vi "SortChannels.vi"(0 "DisplayTetrodes in":refnum<class "DisplayTetrodes.lvclass">, 11 "error in (no error)":errorcluster) -> (1 "sortedTetChanNum":i32[](array[numeric]), 3 "sortedTetNum":i32[](array[numeric]), 4 "DisplayTetrodes out":refnum<class "DisplayTetrodes.lvclass">, 6 "reorderedChanNums":i32[](array[numeric]), 10 "sortedChanIdx":i32[](array[numeric]), 12 "unsortedTetNums":i32[](array[numeric]), 13 "reorderedDiodeChan":i32, 15 "error out":errorcluster)   [LabVIEW 2010, in "DisplayTetrodes.lvclass"]
uses:
  DisplayTetrodes.lvclass
  <vilib>/regexp/Match Regular Expression.xnode
  <vilib>/imath/engines/lvmath2/RunTimeEngine/ErrorHandling/NIMS_Finalize Error.vi
  <vilib>/imath/engines/lvmath2/RunTimeEngine/NodeEndStatement/NIMS_NodeEndStatement_Output.vi
  <instcachedir>/0/NIMS_NodeEndStatement_Output_53EC0D466D134D7ABD903AC30B43404B.lvgen/NIMS_NodeEndStatement_Output_53EC0D466D134D7ABD903AC30B43404B_004.vi
  <instcachedir>/0/NIMS_NodeEndStatement_Output_53EC0D466D134D7ABD903AC30B43404B.lvgen/NIMS_NodeEndStatement_Output_53EC0D466D134D7ABD903AC30B43404B_005.vi
  <instcachedir>/0/NIMS_NodeEndStatement_Output_53EC0D466D134D7ABD903AC30B43404B.lvgen/NIMS_NodeEndStatement_Output_53EC0D466D134D7ABD903AC30B43404B_001.vi
  <vilib>/imath/engines/lvmath2/RunTimeEngine/VariableToken/Read/NIMS_Get Elements - RV(_) - Check(_).vi
  <instcachedir>/0/NIMS_Get Elements - RV(_) - Check(_)_260A45C9C4AF472A8F32F86A1BEF7DEE.lvgen/NIMS_Get Elements - RV(_) - Check(_)_260A45C9C4AF472A8F32F86A1BEF7DEE_001.vi
  <vilib>/imathl/engines/lvmath/Functions/Error Handling/Create Error.vi
  <vilib>/imath/engines/lvmath2/RunTimeEngine/BuiltInFunctions/sort/NIMS_[2o]_sort(RRowV,I32,Str).vi
  <instcachedir>/0/NIMS_[2o]_sort(RRowV,I32,Str)_1834406CABAC430BB40FEC772A4FC192.lvgen/NIMS_[2o]_sort(RRowV,I32,Str)_1834406CABAC430BB40FEC772A4FC192_001.vi
  <vilib>/imath/engines/lvmath2/RunTimeEngine/VariableToken/Read/NIMS_Get Elements - RV(_) - Check.vi
  <instcachedir>/0/NIMS_Get Elements - RV(_) - Check_1F6F8656162345078B1D4DC9877DFAE9.lvgen/NIMS_Get Elements - RV(_) - Check_1F6F8656162345078B1D4DC9877DFAE9_003.vi
  <vilib>/imath/engines/lvmath2/RunTimeEngine/BuiltInFunctions/length/NIMS_length(GV).vi
  <instcachedir>/0/NIMS_length(GV)_08A3D13377FD4E4B96F5795FBF3698FA.lvgen/NIMS_length(GV)_08A3D13377FD4E4B96F5795FBF3698FA_002.vi
  <vilib>/imath/engines/lvmath2/RunTimeEngine/ReplaceToken/NIMS_Replace - Check Linear.vi
  <instcachedir>/0/NIMS_Replace - Check Linear_662D5651E4E34E0584DA82A256193A4C.lvgen/NIMS_Replace - Check Linear_662D5651E4E34E0584DA82A256193A4C_007.vi
  <vilib>/imath/engines/lvmath2/RunTimeEngine/RangeToken/NIMS_Range.vi
  <instcachedir>/0/NIMS_Range_1C63927E4E474DADACDA97C3F2261A11.lvgen/NIMS_Range_1C63927E4E474DADACDA97C3F2261A11_000.vi
  <vilib>/imath/engines/lvmath2/RunTimeEngine/ReplaceToken/NIMS_Replace - Size Check _(_)=VorM.vi
  <instcachedir>/0/NIMS_Replace - Size Check _(_)=VorM_4228B35EE910471DB74F3866D9D09B95.lvgen/NIMS_Replace - Size Check _(_)=VorM_4228B35EE910471DB74F3866D9D09B95_007.vi
  <vilib>/imath/engines/lvmath2/RunTimeEngine/ReplaceToken/NIMS_Replace - Assignment Check _(_)=VorM.vi
  <instcachedir>/0/NIMS_Replace - Assignment Check _(_)=VorM_C130F3B8B64B4DD7B9359A2D3A035D18.lvgen/NIMS_Replace - Assignment Check _(_)=VorM_C130F3B8B64B4DD7B9359A2D3A035D18_007.vi
  <vilib>/imath/engines/lvmath2/RunTimeEngine/ErrorHandling/NIMS_Create Error From Enums.vi
  <vilib>/imath/engines/lvmath2/RunTimeEngine/BuiltInFunctions/findnz/NIMS_[1o]_findnz(GRowV).vi
  <instcachedir>/0/NIMS_[1o]_findnz(GRowV)_005A6E28988F485CA06F579662DA62C7.lvgen/NIMS_[1o]_findnz(GRowV)_005A6E28988F485CA06F579662DA62C7_002.vi
  <vilib>/imath/engines/lvmath2/RunTimeEngine/BuiltInFunctions/is_empty/NIMS_is_empty(GV).vi
  <instcachedir>/0/NIMS_is_empty(GV)_FC7E7C3D9544432CB6AA2416ADCF6D56.lvgen/NIMS_is_empty(GV)_FC7E7C3D9544432CB6AA2416ADCF6D56_000.vi
panel:
  out "size(s) 2":i32
  out "size(s)":i32
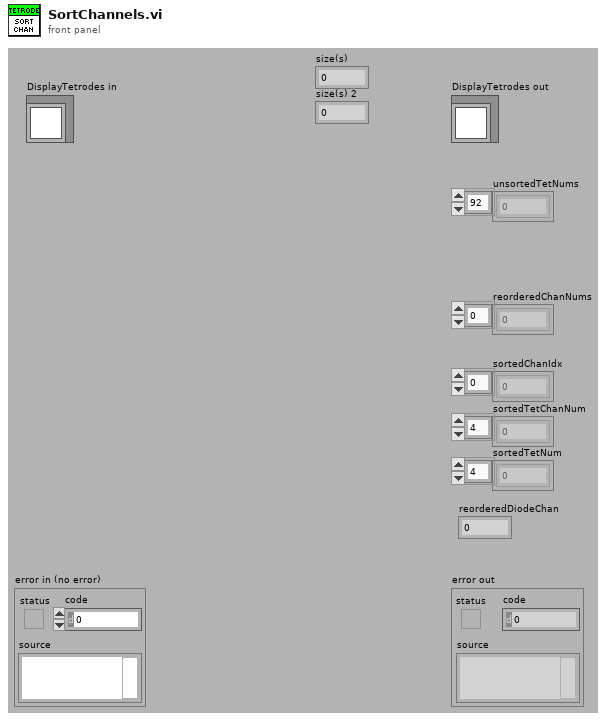
[diagram p1: front panel]
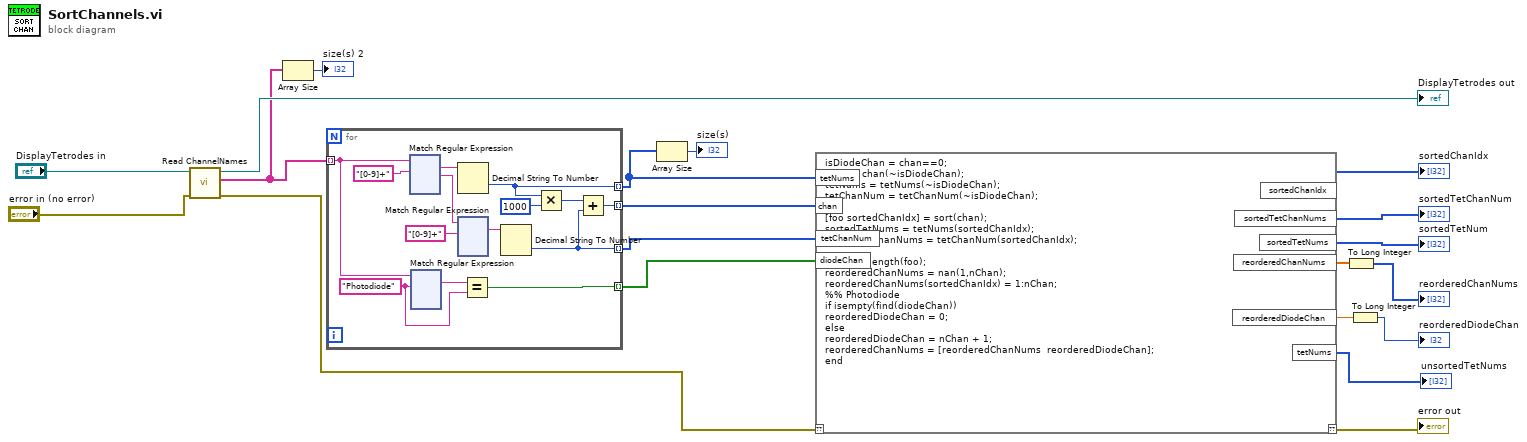
[diagram p0: block diagram]
diagram:
  n1 = call-dynamic "Read ChannelNames.vi"("error in (no error)"="error in (no error)", "DataReceiver in"="DisplayTetrodes in") -> ("error out"=w10:errorcluster, "ChannelNames"=w3:string[], "DataReceiver out"=→"DisplayTetrodes out":refnum<class "DisplayTetrodes.lvclass">)  [unwired: 7 in]
  n2 = Array Size(array=w3) -> (size(s)=→"size(s) 2":i32)
  n3 = for {
    tunnel: w3 -> [w25] mode=indexing
    tunnel: [w22] -> w19 mode=indexing
    tunnel: [w27] -> w5 mode=indexing
    tunnel: [w26] -> w20 mode=indexing
    tunnel: [w21] -> w8 mode=indexing
    w23 = "Photodiode" ("regular expression")
    n4 = xnode "Match Regular Expression"("input string"=w25, "regular expression"="[0-9]+") -> ("whole match"=w31:string, "after match"=w32:string)  [unwired: 4 in, 3 out]
    n5 = xnode "Match Regular Expression"("input string"=w25, "regular expression"=w23) -> ("whole match"=w24:string)  [unwired: 4 in, 4 out]
    n6 = Decimal String To Number(string=w31) -> (number=w27:i32)  [unwired: 2 in, 1 out]
    n7 = xnode "Match Regular Expression"("input string"=w32, "regular expression"="[0-9]+") -> ("whole match"=w30:string)  [unwired: 4 in, 4 out]
    n8 = Equal?(x=w24, y=w23) -> (x = y?=w21:bool)
    n9 = Decimal String To Number(string=w30) -> (number=w26:i32)  [unwired: 2 in, 1 out]
    n10 = Multiply(x=w27, y=1000) -> (x*y=w28:i32)
    n11 = Add(x=w28, y=w26) -> (x+y=w22:i32)
  }
  n12 = Array Size(array=w5) -> (size(s)=→"size(s)":i32)
  n13 = mathscript code="isDiodeChan = chan==0;\nchan = chan(~isDiodeChan);\ntetNums = tetNums(~isDiodeChan);\ntetChanNum = tetChanNum(~isDiodeChan);\n\n[foo sortedChanIdx] = sort(chan);\nsortedTetNums = tetNums(sortedChanIdx);\nsortedTetChanNums = tetChanNum(sortedChanIdx);\n\nnChan = length(foo);\nreorderedChanNums = nan(1,nChan);\nreorderedChanNums(sortedChanIdx) = 1:nChan;\n%% Photodiode\nif isempty(find(diodeChan))\nreorderedDiodeChan = 0;\nelse\nreorderedDiodeChan = nChan + 1;\nreorderedChanNums = [reorderedChanNums  reorderedDiodeChan];\nend"("??"=w10, "chan"=w19, "tetNums"=w5, "tetChanNum"=w20, "diodeChan"=w8) -> ("??"=→"error out":errorcluster, "sortedTetChanNums"=→"sortedTetChanNum":i32[], "sortedTetNums"=→"sortedTetNum":i32[], "sortedChanIdx"=→"sortedChanIdx":i32[], "reorderedChanNums"=w15:dbl[], "reorderedDiodeChan"=w7:dbl, "tetNums"=→"unsortedTetNums":i32[])
  n14 = To Long Integer(number=w15) -> (32bit integer=→"reorderedChanNums":i32[])
  n15 = To Long Integer(number=w7) -> (32bit integer=→"reorderedDiodeChan":i32)
